vi "Luefter neue Version.vi"(10 "Lüfter":sgl, 11 "Schaltschranktemp.":sgl) -> ()   [LabVIEW 2020, in "Allgemein.lvlib"]
uses:
  Allgemein.lvlib
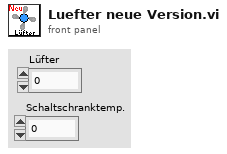
[diagram p1: front panel]
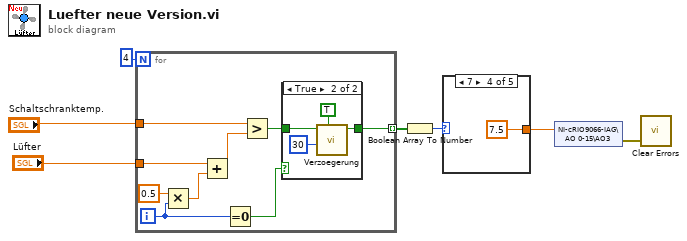
[diagram p0: block diagram]
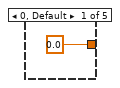
[diagram p2: hidden frame]
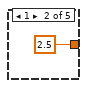
[diagram p3: hidden frame]
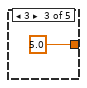
[diagram p4: hidden frame]
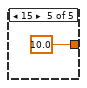
[diagram p5: hidden frame]
diagram:
  n1 = for {
    N: 4 -> [_]
    tunnel: "Schaltschranktemp." -> [w15]
    tunnel: [w10] -> w6 mode=indexing
    tunnel: "Lüfter" -> [w16]
    i -> [w9]
    n2 = Multiply(x=sgl 0.5 ("y"), y=w9) -> (x*y=w12:sgl)
    n3 = Add(x=w16, y=w12) -> (x+y=w14:sgl)
    n4 = Equal To 0?(x=w9) -> (x = 0?=w8:bool)
    n5 = Greater?(x=w15, y=w14) -> (0:w11:bool)
    n6 = case shown="True" w8 {
      tunnel: w11 -> [w17 w19]
      tunnel: [w17 w18] -> w10
      frame False {
      }
      frame True {
        n7 = call "Verzoegerung.vi"("Abfallverzögerung?"=TRUE, "sec"=u16 30, "Startsignal"=w19) -> ("Zeit abgelaufen?"=w18:bool)  [unwired: 7 in, 1 out]
      }
    }
  }
  n8 = Boolean Array To Number(Boolean array=w6) -> (number=w3:u32)
  n9 = case shown="7" w3 {
    tunnel: [0.0 2.5 5.0 7.5 10.0] -> w1
    frame 0, Default {
    }
    frame 1 {
    }
    frame 3 {
    }
    frame 7 {
    }
    frame 15 {
    }
  }
  n10 = shared-variable "NI-cRIO9066-IAG\\AO 0-15\\AO3"(w1) -> (error out=w2:errorcluster)  [unwired: 1 in]
  n11 = call <vilib>:"Clear Errors.vi"("error in (no error)"=w2) -> ()  [unwired: 5 in, 2 out]
